vi "default_phase.vi"(9 "dimension size y":i32, 10 "dimension size x":i32, 11 "frekanslar":dbl[](array[numeric])) -> (3 "R/P Array":dbl[][](array[numeric]))   [LabVIEW 2014]
panel:
  in  "hz title array":dbl[](array[numeric])
  in  "Tbl Refnum":refnum<vi>
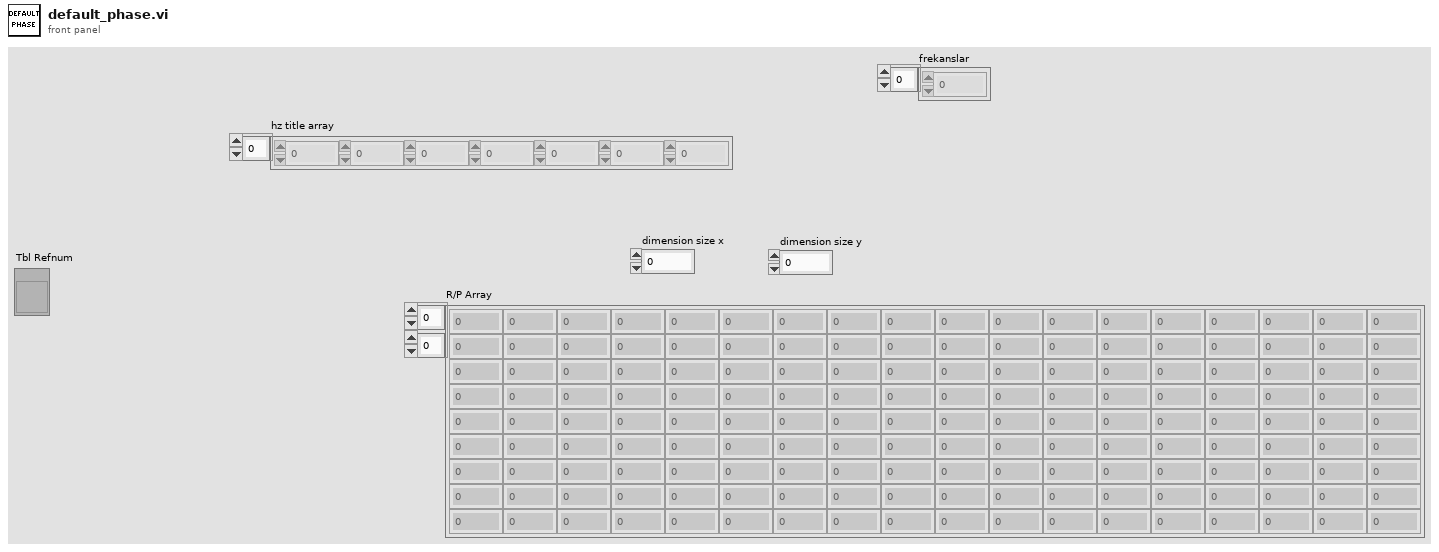
[diagram p1: front panel]
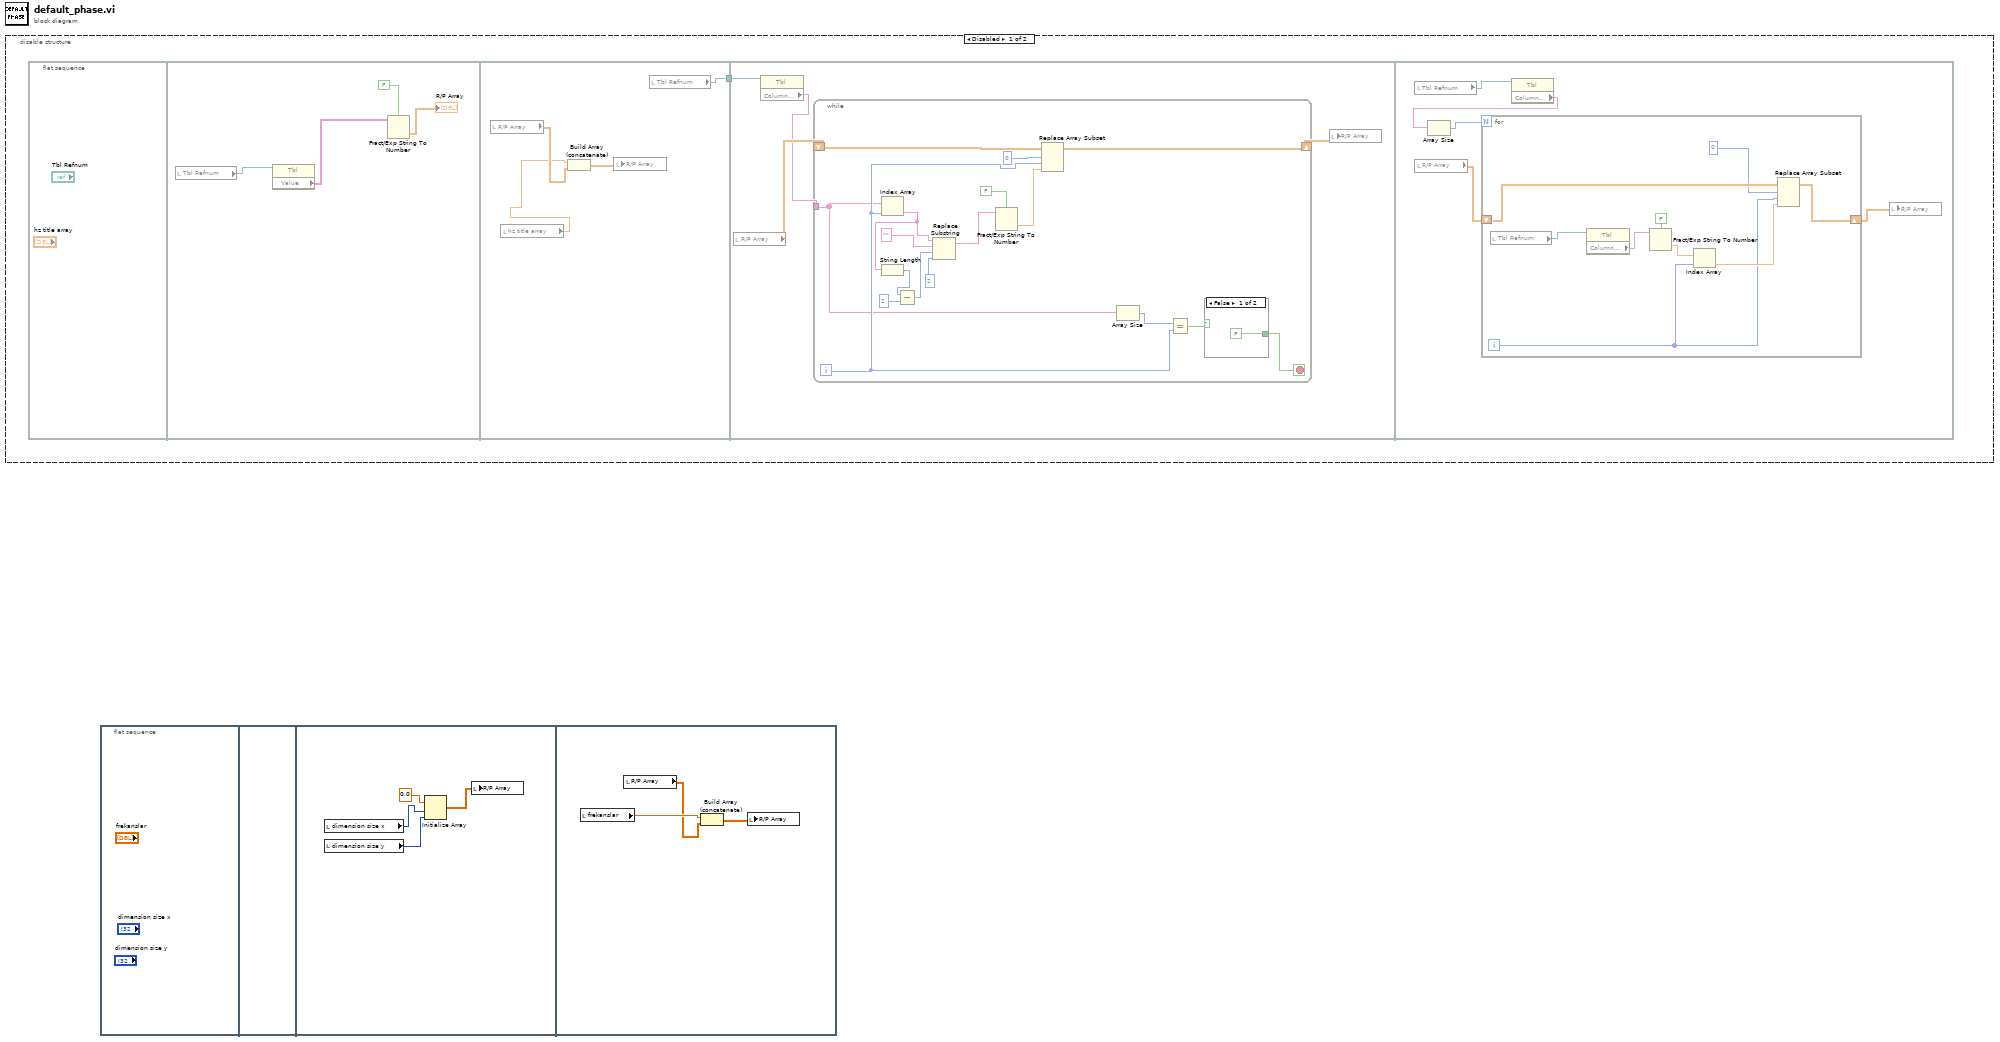
[diagram p0: block diagram]
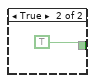
[diagram p2: hidden frame]
diagram:
  n1 = disable-structure shown="Disabled" {
    frame Disabled {
      n2 = flat-sequence {
        tunnel: [w7] -> w1
        tunnel: w1 -> [w11]
        frame #0 {
        }
        frame #1 {
          n3 = local read "Tbl Refnum"() -> (w5:refnum<vi>)
          n4 = property class="Tbl"(reference=w5) -> ("Value"=w3:string[][])  [unwired: 1 in, 2 out]
          n5 = Fract/Exp String To Number(use system decimal point (T)=FALSE, string=w3) -> (number=→"R/P Array":dbl[][])  [unwired: 2 in, 1 out]
        }
        frame #2 {
          n6 = local read "R/P Array"() -> (w8:dbl[][])
          n7 = local read "hz title array"() -> (w6:dbl[])
          n8 = Build Array (concatenate)(w6, w8) -> (w9:dbl[][])
          n9 = local write "R/P Array"(w9) -> ()
          n10 = local read "Tbl Refnum"() -> (w7:refnum<vi>)
        }
        frame #3 {
          n11 = local read "R/P Array"() -> (w13:dbl[][])
          n12 = property class="Tbl"(reference=w11) -> ("Column Headers[]"=w10:string[])  [unwired: 1 in, 2 out]
          n13 = while {
            tunnel: w10 -> [w15]
            shift-right: [w19] -> w12
            shift-left: w13 -> [w20]
            i -> [w17]
            stop <- w14 stop-if-true
            n14 = Index Array(array=w15, index=w17) -> (element=w26:string)
            n15 = String Length(string=w26) -> (length=w28:i32)
            n16 = Subtract(x=w28, y=2) -> (x-y=w25:i32)
            n17 = Replace Substring(2:2 ("length (len. of substring)"), 3:w25, 4:"" ("substring (\"\")"), 5:w26) -> (1:w23:string)  [unwired: 1 out]
            n18 = Fract/Exp String To Number(use system decimal point (T)=FALSE, string=w23) -> (number=w21:dbl)  [unwired: 2 in, 1 out]
            n19 = Replace Array Subset(array=w20, new element=w21, index (row)=0, index (col)=w17) -> (w19:dbl[][])
            n20 = Array Size(array=w15) -> (size(s)=w16:i32)
            n21 = Equal?(x=w16, y=w17) -> (x = y?=w18:bool)
            n22 = case shown="False" w18 {
              tunnel: [FALSE TRUE] -> w14
              frame False {
              }
              frame True {
              }
            }
          }
          n23 = local write "R/P Array"(w12) -> ()
        }
        frame #4 {
          n24 = local read "Tbl Refnum"() -> (w35:refnum<vi>)
          n25 = local read "R/P Array"() -> (w37:dbl[][])
          n26 = property class="Tbl"(reference=w35) -> ("Column Headers[]"=w34:string[])  [unwired: 1 in, 2 out]
          n27 = Array Size(array=w34) -> (size(s)=w33:i32)
          n28 = for {
            N: w33 -> [_]
            shift-right: [w45] -> w36
            shift-left: w37 -> [w46]
            i -> [w38]
            n29 = local read "Tbl Refnum"() -> (w42:refnum<vi>)
            n30 = property class="Tbl"(reference=w42) -> ("Column Headers[]"=w44:string[])  [unwired: 1 in, 2 out]
            n31 = Fract/Exp String To Number(use system decimal point (T)=FALSE, string=w44) -> (number=w41:dbl[])  [unwired: 2 in, 1 out]
            n32 = Index Array(array=w41, index=w38) -> (element=w39:dbl)
            n33 = Replace Array Subset(array=w46, new element=w39, index (row)=0 ("disabled index (row)"), index (col)=w38) -> (w45:dbl[][])
          }
          n34 = local write "R/P Array"(w36) -> ()
        }
      }
    }
    frame Enabled {
    }
  }
  n35 = flat-sequence {
    frame #0 {
    }
    frame #1 {
    }
    frame #2 {
      n36 = local read "dimension size x"() -> (w49:i32)
      n37 = local read "dimension size y"() -> (w50:i32)
      n38 = Initialize Array(0.0 ("element"), w49, w50) -> (w47:dbl[][])
      n39 = local write "R/P Array"(w47) -> ()
    }
    frame #3 {
      n40 = local read "frekanslar"() -> (w53:dbl[])
      n41 = local read "R/P Array"() -> (w51:dbl[][])
      n42 = Build Array (concatenate)(w53, w51) -> (w52:dbl[][])
      n43 = local write "R/P Array"(w52) -> ()
    }
  }
